vi "Get Relative Sizes.vi"(8 "error in (no error)":errorcluster, 11 "Divider in":refnum<class "Divider.lvclass">) -> (0 "error out":errorcluster, 2 "Relative sizes":dbl[](array[numeric]), 3 "Divider out":refnum<class "Divider.lvclass">)   [LabVIEW 2021, in "Divider.lvclass"]
doc: "Copyright 2018, Wiebe Walstra, wiebe@carya.nl."
uses:
  Divider.lvclass
  Divider.lvclass/Divider.ctl
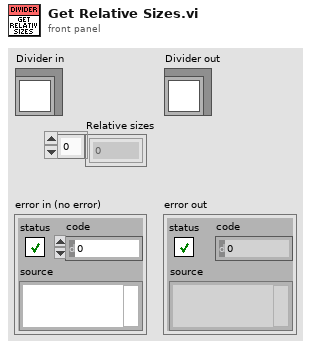
[diagram p1: front panel]
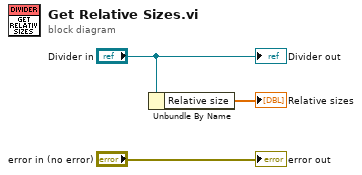
[diagram p0: block diagram]
diagram:
  n1 = Unbundle By Name("Divider in") -> ("Relative size"=→"Relative sizes":dbl[])
  "error out" <- "error in (no error)"
  "Divider out" <- "Divider in"
